vi "Read RFPM Session.vi"(8 "error in (no error)":errorcluster, 11 "Vector Path in":refnum<class "Vector 18GHz Path.lvclass">) -> (0 "error out":errorcluster, 2 "RFPM Session":refnum<k15>, 3 "Vector Path out":refnum<class "Vector 18GHz Path.lvclass">)   [LabVIEW 2023, in "RFFixtureCharact.RFPM.lvlib" / "Vector 18GHz Path.lvclass"]
uses:
  Vector 18GHz Path.lvclass
  Vector 18GHz Path.lvclass/Vector 18GHz Path.ctl
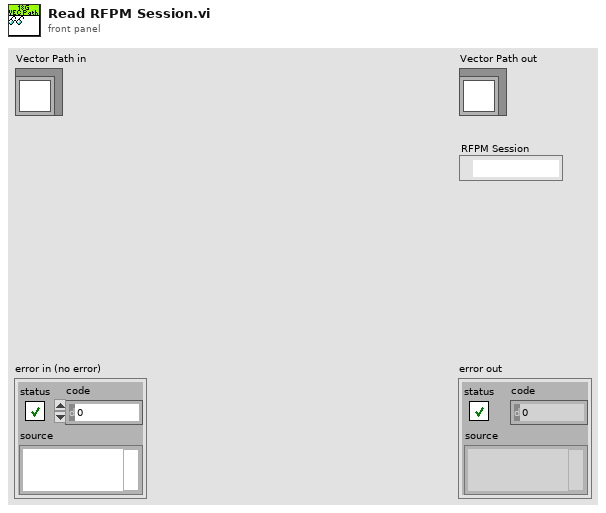
[diagram p1: front panel]
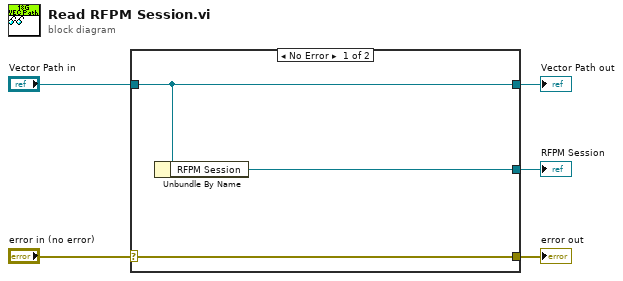
[diagram p0: block diagram]
diagram:
  n1 = case shown="No Error" "error in (no error)" {
    selector: "error in (no error)" -> [w8 w9]
    tunnel: [w8 w9] -> w4
    tunnel: [w7 w10] -> w2
    tunnel: "Vector Path in" -> [w7 w10]
    tunnel: [w6 _] -> w1
    frame No Error {
      n2 = Unbundle By Name(w7) -> ("RFPM Session"=w6:refnum<k15>)
    }
    frame Error {
    }
  }
  "error out" <- w4
  "Vector Path out" <- w2
  "RFPM Session" <- w1
